vi "BATTERY AVAILABLE ENERGY VI.vi"(0 "unsigned byte array[7]":u8, 1 "unsigned byte array[6]":u8, 2 "unsigned byte array[5]":u8, 3 "unsigned byte array[1]":u8, 5 "unsigned byte array[8]":u8, 7 "Numeric 4":dbl, 9 "Numeric 3":dbl, 11 "Numeric 5":dbl, 12 "Boolean":bool, 13 "Numeric 2":dbl, 14 "Numeric":dbl) -> (4 "Numeric 9":dbl, 6 "Numeric 8":dbl, 8 "Numeric 7":dbl, 10 "Numeric 6":dbl, 15 "Numeric 10":dbl)   [LabVIEW 2016]
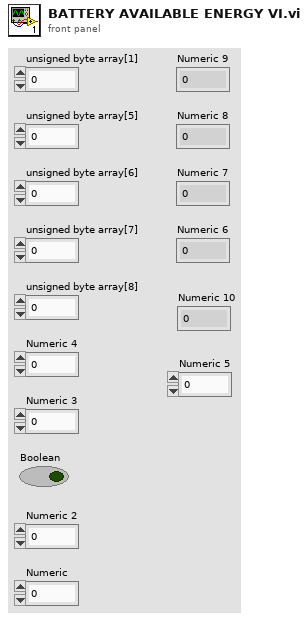
[diagram p1: front panel]
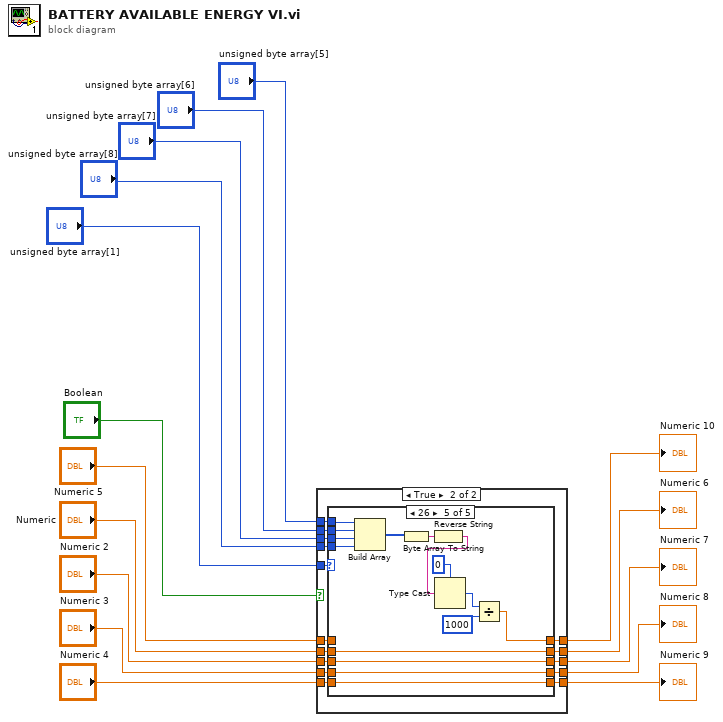
[diagram p0: block diagram]
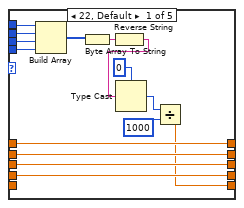
[diagram p3: hidden frame]
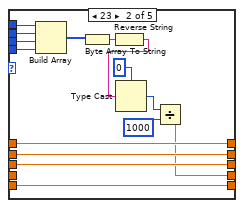
[diagram p4: hidden frame]
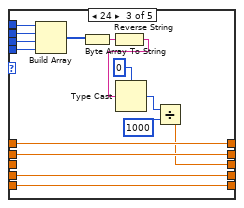
[diagram p5: hidden frame]
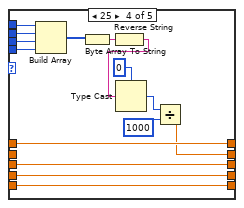
[diagram p6: hidden frame]
diagram:
  n1 = case shown="True" "Boolean" {
    tunnel: "unsigned byte array[5]" -> [_ w36]
    tunnel: "unsigned byte array[6]" -> [_ w35]
    tunnel: "unsigned byte array[7]" -> [_ w34]
    tunnel: "unsigned byte array[8]" -> [_ w33]
    tunnel: "unsigned byte array[1]" -> [_ w32]
    tunnel: [w17 w31] -> w11
    tunnel: "Numeric 4" -> [w17 w30]
    tunnel: "Numeric 3" -> [w18 w29]
    tunnel: [w18 w28] -> w8
    tunnel: "Numeric 2" -> [w19 w27]
    tunnel: [w19 w26] -> w6
    tunnel: "Numeric" -> [w20 w25]
    tunnel: [w20 w24] -> w4
    tunnel: "Numeric 5" -> [w21 w23]
    tunnel: [w21 w22] -> w2
    frame False {
    }
    frame True {
      n2 = case shown="26" w32 {
        tunnel: w36 -> [w45 w60 w75 w90 w105]
        tunnel: w35 -> [w44 w59 w74 w89 w104]
        tunnel: w34 -> [w43 w58 w73 w88 w103]
        tunnel: w33 -> [w42 w57 w72 w87 w102]
        tunnel: [w37 w56 w70 w85 w100] -> w31
        tunnel: w30 -> [_ w56 w70 w85 w100]
        tunnel: w29 -> [w41 _ w71 w86 w101]
        tunnel: [w41 w52 w71 w86 w101] -> w28
        tunnel: [w40 w55 w67 w84 w99] -> w26
        tunnel: w27 -> [w40 w55 _ w84 w99]
        tunnel: [w39 w54 w69 w82 w98] -> w24
        tunnel: w25 -> [w39 w54 w69 _ w98]
        tunnel: [w38 w53 w68 w83 w97] -> w22
        tunnel: w23 -> [w38 w53 w68 w83 _]
        frame 22, Default {
          n3 = Build Array(w45, w44, w43, w42) -> (w51:u8[])
          n4 = Byte Array To String(unsigned byte array=w51) -> (string=w50:string)
          n5 = Reverse String(1:w50) -> (0:w46:string)
          n6 = Type Cast(type=0, x=w46) -> (*(type *) &x=w48:i32)
          n7 = Divide(x=w48, y=1000) -> (x/y=w37:dbl)
        }
        frame 23 {
          n8 = Build Array(w60, w59, w58, w57) -> (w66:u8[])
          n9 = Byte Array To String(unsigned byte array=w66) -> (string=w65:string)
          n10 = Reverse String(1:w65) -> (0:w61:string)
          n11 = Type Cast(type=0, x=w61) -> (*(type *) &x=w63:i32)
          n12 = Divide(x=w63, y=1000) -> (x/y=w52:dbl)
        }
        frame 24 {
          n13 = Build Array(w75, w74, w73, w72) -> (w81:u8[])
          n14 = Byte Array To String(unsigned byte array=w81) -> (string=w80:string)
          n15 = Reverse String(1:w80) -> (0:w76:string)
          n16 = Type Cast(type=0, x=w76) -> (*(type *) &x=w78:i32)
          n17 = Divide(x=w78, y=1000) -> (x/y=w67:dbl)
        }
        frame 25 {
          n18 = Build Array(w90, w89, w88, w87) -> (w96:u8[])
          n19 = Byte Array To String(unsigned byte array=w96) -> (string=w95:string)
          n20 = Reverse String(1:w95) -> (0:w91:string)
          n21 = Type Cast(type=0, x=w91) -> (*(type *) &x=w93:i32)
          n22 = Divide(x=w93, y=1000) -> (x/y=w82:dbl)
        }
        frame 26 {
          n23 = Build Array(w105, w104, w103, w102) -> (w111:u8[])
          n24 = Byte Array To String(unsigned byte array=w111) -> (string=w110:string)
          n25 = Reverse String(1:w110) -> (0:w106:string)
          n26 = Type Cast(type=0, x=w106) -> (*(type *) &x=w108:i32)
          n27 = Divide(x=w108, y=1000) -> (x/y=w97:dbl)
        }
      }
    }
  }
  "Numeric 6" <- w4
  "Numeric 7" <- w6
  "Numeric 8" <- w8
  "Numeric 9" <- w11
  "Numeric 10" <- w2
